vi "PH_AWG-510.PC Set Trigger Settings.vi"(0 "VI in":refnum<vi>, 2 "Wanted Trigger Settings":T1, 5 "error in (no error)":errorcluster) -> (14 "VI out":refnum<vi>, 19 "error out":errorcluster)   [LabVIEW 2014, in "PH_AWG-510.lvlib"]
doc: "This VI sets the trigger settings of the hardware and requests afterwards the current settings to store them on own attributes and to display them at the GUI."
uses:
  PH_AWG-510.lvlib
  PH_AWG-510.Trigger Settings.ctl
  instr.lib/awg510/Tektronix AWG510.lvlib
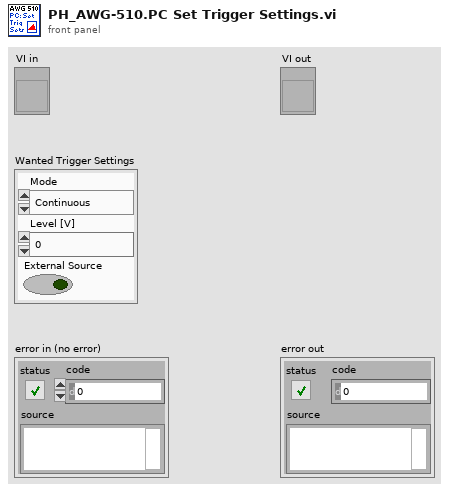
[diagram p1: front panel]
types:
  T1 = typedef "PH_AWG-510.lvlib/PH_AWG-510.Trigger Settings.ctl" = cluster{"Mode":enum16{"Continuous", "Triggered", "Gated", "Enhanced"}, "Level (V)":dbl, "External Source":bool}
  T2 = typedef "PH_AWG-510.lvlib/PH_AWG-510.i attribute.ctl" = cluster{"GUI Refs":cluster{"Delete":refnum<vi>, "Trigger Settings":refnum<vi>, "Start Device":refnum<vi>, "Instrument Information":refnum<vi>, "Lock Frontpanel":refnum<vi>, "Waveform Pattern File":refnum<vi>, "Initialize":refnum<vi>, "Output Settings":refnum<vi>}, "Instrument Information":T3, "Initialized?":bool, "Current Settings":cluster{"Trigger":T1, "Output Settings":T4}, "Wanted Settings":cluster{"Trigger":T1, "Output Settings":T4}, "Device frontpanel locked?":bool, "Default File Path":path}
  T3 = typedef "PH_AWG-510.lvlib/PH_AWG-510.Instrument Information Dataset.ctl" = cluster{"VISA resource name":refnum<visa-resource-name>, "Instrument Firmware Revision":string, "Manufacturer":string, "Model":string, "Serial Number":string, "Error Message":string, "Device Status":enum16{"stopped", "wating for trigger", "running", "Failure"}}
  T4 = typedef "PH_AWG-510.lvlib/PH_AWG-510.Output Settings.ctl" = cluster{"Activate Channel":bool, "VPP (V)":dbl, "Clock (Hz)":dbl, "File Name (Device)":string, "#1":u16, "#2":u16, "#3":u16, "#4":u16, "#5":u16, "#6":u16, "#7":u16, "#8":u16, "#9":u16, "#10":u16, "#11":u16, "#12":u16, "#13":u16, "#14":u16, "#15":u16, "#16":u16, "#17":u16, "#18":u16, "#19":u16, "#20":u16, "Offset (V)":dbl}
  T5 = enum16{"Continuous", "Triggered", "Gated", "Enhanced"}
  T6 = enum8{"Enabled", "Disabled", "Disabled and Grayed Out"}
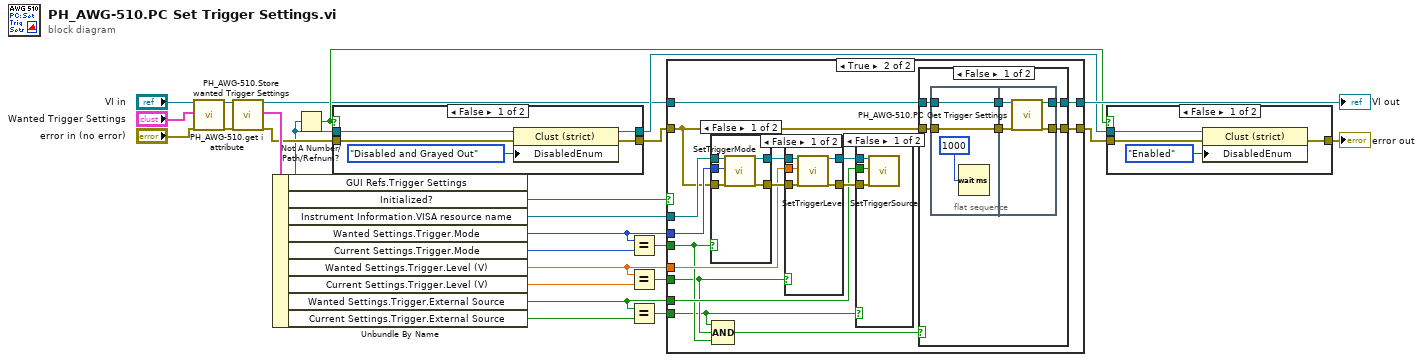
[diagram p0: block diagram]
diagram:
  n1 = call "PH_AWG-510.Store wanted Trigger Settings.vi"("VI in"="VI in", "Wanted Trigger Settings"="Wanted Trigger Settings", "error in (no error)"="error in (no error)") -> ("VI out"=w6:refnum<vi>, "error out"=w5:errorcluster)  [unwired: 15 in]
  n2 = call "PH_AWG-510.get i attribute.vi"("i ref in"=w6, "error in (no error)"=w5) -> ("i ref out"=w2:refnum<vi>, "i attribute"=w26:T2, "error out"=w12:errorcluster)  [unwired: 15 in]
  n3 = Unbundle By Name(w26) -> ("GUI Refs.Trigger Settings"=w10:refnum<vi>, "Initialized?"=w18:bool, "Instrument Information.VISA resource name"=w22:refnum<visa-resource-name>, "Wanted Settings.Trigger.Mode"=w21:T5, "Current Settings.Trigger.Mode"=w25:T5, "Wanted Settings.Trigger.Level (V)"=w20:dbl, "Current Settings.Trigger.Level (V)"=w24:dbl, "Wanted Settings.Trigger.External Source"=w19:bool, "Current Settings.Trigger.External Source"=w23:bool)
  n4 = Not A Number/Path/Refnum?(number/path/refnum=w10) -> (NaN/Path/Refnum?=w9:bool)
  n5 = case shown="False" w9 {
    tunnel: w12 -> [w31 w33]
    tunnel: [w30 w33] -> w1
    tunnel: w10 -> [w29 w32]
    tunnel: [w27 w32] -> w11
    frame False {
      n6 = property class="Clust (strict)"(reference=w29, error in=w31, "DisabledEnum"=T6."Disabled and Grayed Out" ("Disabled")) -> (reference out=w27:refnum<vi>, error out=w30:errorcluster)
    }
    frame True {
    }
  }
  n7 = Equal?(x=w21, y=w25) -> (x = y?=w17:bool)
  n8 = Equal?(x=w20, y=w24) -> (x = y?=w15:bool)
  n9 = Equal?(x=w19, y=w23) -> (x = y?=w16:bool)
  n10 = case shown="True" w18 {
    tunnel: w22 -> [_ w49]
    tunnel: w21 -> [_ w46]
    tunnel: w20 -> [_ w45]
    tunnel: w19 -> [_ w44]
    tunnel: w17 -> [_ w43]
    tunnel: w16 -> [_ w41]
    tunnel: w15 -> [_ w42]
    tunnel: w1 -> [w34 w36]
    tunnel: w2 -> [w35 w40]
    tunnel: [w35 w39] -> w14
    tunnel: [w34 w38] -> w8
    frame False {
    }
    frame True {
      n11 = case shown="False" w43 {
        tunnel: [w81 w82] -> w51
        tunnel: w49 -> [w80 w83]
        tunnel: [w79 w83] -> w48
        tunnel: w36 -> [w78 w82]
        tunnel: w46 -> [w77 _]
        frame False {
          n12 = call "SetTriggerMode.vi"("VISA resource name"=w80, "Trigger Mode"=w77, "error in"=w78) -> ("VISA resource name out"=w79:refnum<visa-resource-name>, "error out"=w81:errorcluster)  [unwired: 15 in]
        }
        frame True {
        }
      }
      n13 = Compound Arithmetic op=AND(w41, w42, w43) -> (w37:bool)
      n14 = case shown="False" w42 {
        tunnel: w51 -> [w74 w75]
        tunnel: [w73 w75] -> w50
        tunnel: w48 -> [w72 w76]
        tunnel: [w71 w76] -> w47
        tunnel: w45 -> [w70 _]
        frame False {
          n15 = call "SetTriggerLevel.vi"("VISA resource name"=w72, "Trigger Level (V)"=w70, "error in"=w74) -> ("VISA resource name out"=w71:refnum<visa-resource-name>, "error out"=w73:errorcluster)  [unwired: 15 in]
        }
        frame True {
        }
      }
      n16 = case shown="False" w41 {
        tunnel: w50 -> [w69 _]
        tunnel: w47 -> [w68 _]
        tunnel: w44 -> [w67 _]
        frame False {
          n17 = call "SetTriggerSource.vi"("VISA resource name"=w68, "Trigger source external? (false)"=w67, "error in"=w69) -> ()  [unwired: 15 in, 2 out]
        }
        frame True {
        }
      }
      n18 = case shown="False" w37 {
        tunnel: w36 -> [w57 w65]
        tunnel: [w56 w65] -> w38
        tunnel: w40 -> [w55 w66]
        tunnel: [w54 w66] -> w39
        frame False {
          n19 = flat-sequence {
            tunnel: w55 -> [w59]
            tunnel: w57 -> [w60]
            tunnel: [w60] -> w53
            tunnel: [w59] -> w52
            tunnel: [w63] -> w56
            tunnel: [w61] -> w54
            tunnel: w53 -> [w64]
            tunnel: w52 -> [w62]
            frame #0 {
              n20 = Wait (ms)(milliseconds to wait=u32 1000) -> ()  [unwired: 1 out]
            }
            frame #1 {
              n21 = call "PH_AWG-510.PC Get Trigger Settings.vi"("VI in"=w62, "error in (no error)"=w64) -> ("VI out"=w61:refnum<vi>, "error out"=w63:errorcluster)  [unwired: 16 in]
            }
          }
        }
        frame True {
        }
      }
    }
  }
  "VI out" <- w14
  n22 = case shown="False" w9 {
    tunnel: w8 -> [w87 w88]
    tunnel: [w86 w88] -> w7
    tunnel: w11 -> [w85 _]
    frame False {
      n23 = property class="Clust (strict)"(reference=w85, error in=w87, "DisabledEnum"=T6."Enabled" ("Disabled")) -> (error out=w86:errorcluster)  [unwired: 1 out]
    }
    frame True {
    }
  }
  "error out" <- w7
